vi "LDT1001 Getting Started.vi"(7 "RS485 Addr. (128: RS232)":u32=128 max=128, 9 "Reset / Default (T: Both)":bool=TRUE, 10 "ID Query (T: Check)":bool=TRUE, 11 "Serial Port (Com 1: Default)":u16(ring) items=["Com 1", "Com 2", "Com 3", "Com 4"]) -> (0 "error out":errorcluster, 2 "Instrument Identity":string)   [LabVIEW 2011]
doc: "This VI demonstrates the general use of the instrument VIs. It should operate properly with all series of instruments, namely E2xx, E3xx (new and older revisions), RE3xx and Integra. Since this VI checks for functions supported with every of the instruments, no serious problems should appear.\n\nOnly two instrument dependent errors may appear: 1) if an external circuit is supported but no external sensor is present, 2) if a refrigerator level (i.e. 2) is used, that is not valid for the type of instrument used. For Series Integra automatically the refrigerator level and the pump power level settings are ignored by this Getting started VI.\n\nAll other errors, that may appear, are communication errors.\n\nSo, on any errors, check for proper settings of the communication port, the baudrate and/or the correct RS485 address (or 128 for RS232 communication) first."
panel:
  out "Ramp Programs Message":string="Max. Count of Ramp Programs and Segments is:"
  out "Max. Segment Count":u8
  out "Ramps available":u8
  out "Pump Pressure is (Integra only)":dbl format="%.2f"
  out "External Bath Temperature is:":dbl format="%.2f"
  out "PID Value P/°C":dbl format="%.2f"
  out "PID Value I/s":i32
  out "Upper Temperature":dbl format="%.2f"
  out "Lower Temperature":dbl format="%.2f"
  out "Ext. Circuit Message":string="External Circuit Settings are:"
  out "Error Status Word":string
  out "Software Rev.":string
  out "Hardware Rev.":string
  out "Self-Test":string
  out "Support Message":string="Pump Power / Refrigerator Levels are:"
  in  "Baud Rate (2: 9600 Default)":u16(ring)=2 items=["2400", "4800", "9600", "19200"]
  out "Serial Port":string
  out "PID Value I/s":i32
  out "PID Value P/°C":dbl format="%.2f"
  out "Pump Power Level":u8
  out "Refrigerator Level":u8
  out "Cutoff/°C":dbl format="%.2f"
  out "Bath temperature/°C":dbl format="%.2f"
  out "Setpoint/°C":dbl format="%.2f"
  in  "Setpoint/°C (20.00 °C: Default)":sgl=20.0 min=-35 max=250 step=1 format="%.2f"
  in  "Refrigerator Level (0: Default)":u8 max=3
  in  "Pump Power Level (2: Default)":u8=1 min=1 max=5
  out "Error Message":string="No Error"
  # "Getting Started"
  # "Settings"
  # "Readings"
  # "Communication"
  # "Instrument"
  # "Outlet Temperature Values are:"
  # "Temperature (Primary Circuit Settings) are:"
  # "PID Values External are:"
  # "Check\nDon't Check"
  # "Reset and Default\nDefault only"
  # "PID Values Internal are:"
  # "Instrument"
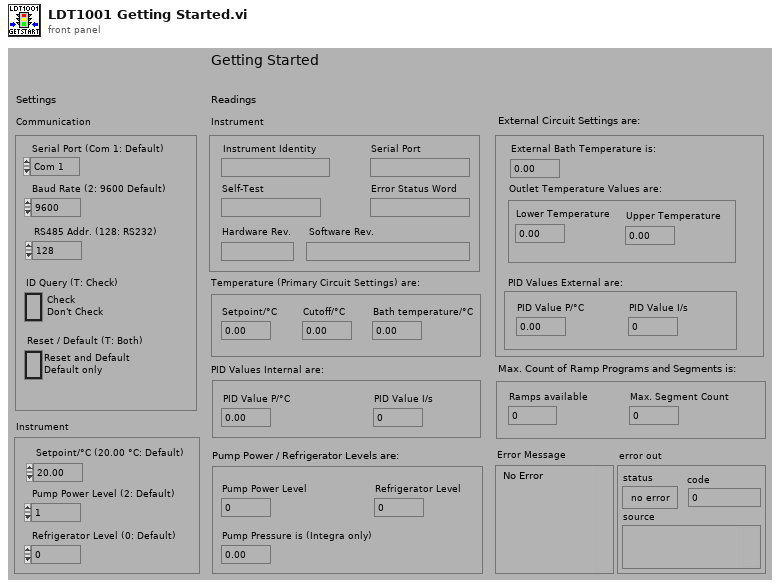
[diagram p1: front panel]
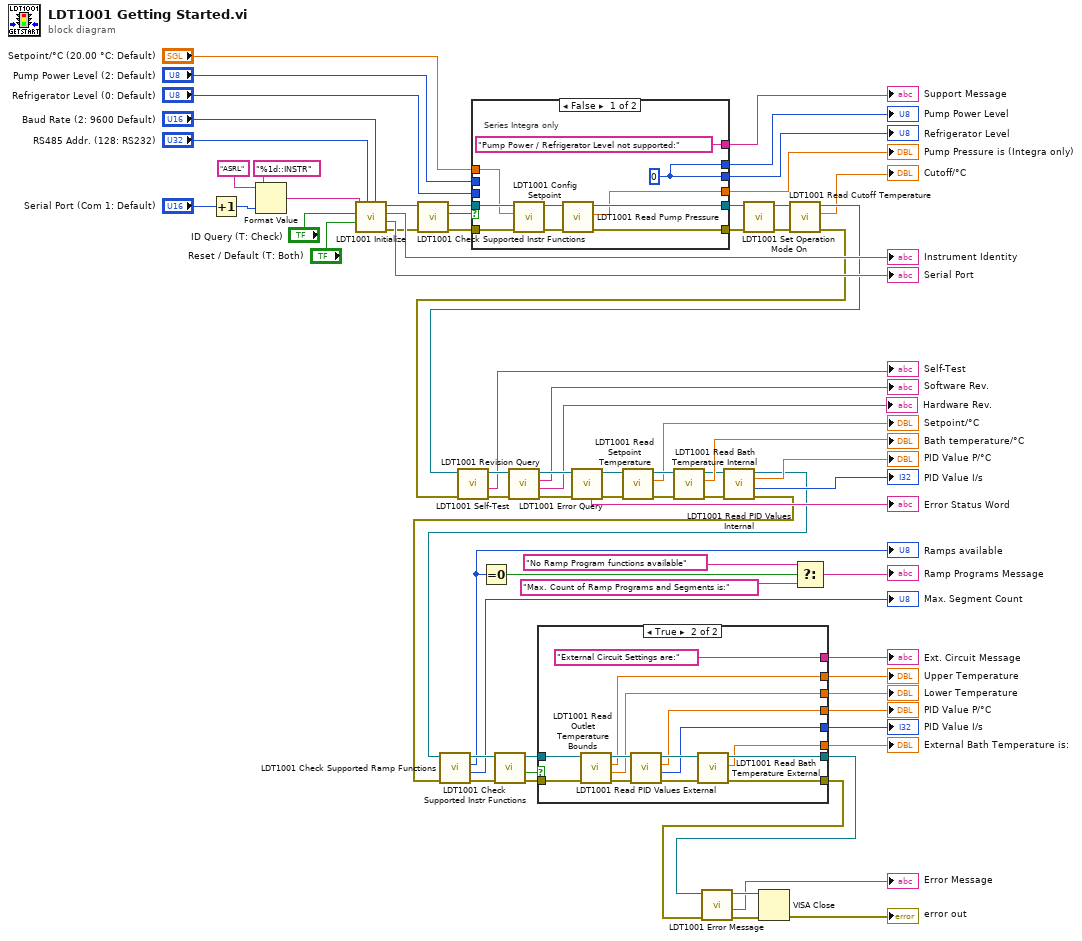
[diagram p0: block diagram]
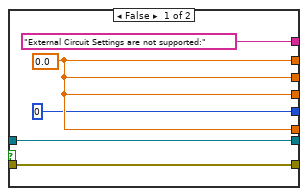
[diagram p2: hidden frame]
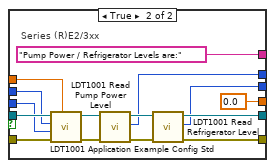
[diagram p3: hidden frame]
diagram:
  n1 = Increment(x="Serial Port (Com 1: Default)") -> (x+1=w53:u16)
  n2 = Format Value(string ("")="ASRL", format string="%1d::INSTR", value (0)=w53) -> (output string=w56:string)
  n3 = call <instrlib>:"LDT1001 Initialize.vi"("Baud Rate (2: 9600 default)"="Baud Rate (2: 9600 Default)", "RS485 Instrument Address (128: RS232 default)"="RS485 Addr. (128: RS232)", "Reset / Default (T: Both)"="Reset / Default (T: Both)", "ID Query (T: Check)"="ID Query (T: Check)", "Instrument Descriptor (ASRL1::INSTR)"=w56) -> ("error out"=w46:errorcluster, "Serial Port"=→"Serial Port":string, "Instrument Identity"=→"Instrument Identity":string, "VISA session"=w47:refnum<visa-resource-name>)  [unwired: 3 in]
  n4 = call <instrlib>:"LDT1001 Check Supported Instr Functions.vi"("error in (no error)"=w46, "VISA session"=w47) -> ("error out"=w49:errorcluster, "Pump/Refrig supported"=w45:bool, "dup VISA session"=w48:refnum<visa-resource-name>)  [unwired: 6 in, 1 out]
  n5 = case shown="False" w45 {
    tunnel: w48 -> [w83 w98]
    tunnel: w49 -> [w82 w97]
    tunnel: [w75 w89] -> w50
    tunnel: [w76 w88] -> w51
    tunnel: "Refrigerator Level (0: Default)" -> [_ w96]
    tunnel: "Pump Power Level (2: Default)" -> [_ w95]
    tunnel: "Setpoint/°C (20.00 °C: Default)" -> [w81 w94]
    tunnel: [w79 w87] -> w41
    tunnel: [w79 w86] -> w65
    tunnel: ["Pump Power / Refrigerator Level not supported:" "Pump Power / Refrigerator Levels are:"] -> w40
    tunnel: [w74 0.0] -> w13
    frame False {
      w79 = u8 0
      # "Series Integra only"
      n6 = call <instrlib>:"LDT1001 Config Setpoint.vi"("error in (no error)"=w82, "Setpoint (20.00 °C: Default)"=w81, "VISA session"=w83) -> ("error out"=w78:errorcluster, "dup VISA session"=w77:refnum<visa-resource-name>)  [unwired: 7 in]
      n7 = call <instrlib>:"LDT1001 Read Pump Pressure.vi"("error in (no error)"=w78, "VISA session"=w77) -> ("error out"=w75:errorcluster, "Pump Pressure"=w74:dbl, "dup VISA session"=w76:refnum<visa-resource-name>)  [unwired: 7 in]
    }
    frame True {
      # "Series (R)E2/3xx"
      n8 = call <instrlib>:"LDT1001 Application Example Config Std.vi"("Setpoint (20.00 °C: Default)"=w94, "error in (no error)"=w97, "Refrigerator Level (0: Default)"=w96, "Pump Power Level (2: Default)"=w95, "VISA session"=w98) -> ("error out"=w90:errorcluster, "dup VISA session"=w92:refnum<visa-resource-name>)  [unwired: 5 in]
      n9 = call <instrlib>:"LDT1001 Read Pump Power Level.vi"("error in (no error)"=w90, "VISA session"=w92) -> ("error out"=w91:errorcluster, "Pump Power Level"=w86:u8, "dup VISA session"=w93:refnum<visa-resource-name>)  [unwired: 7 in]
      n10 = call <instrlib>:"LDT1001 Read Refrigerator Level.vi"("error in (no error)"=w91, "VISA session"=w93) -> ("error out"=w89:errorcluster, "Refrigerator Level"=w87:u8, "dup VISA session"=w88:refnum<visa-resource-name>)  [unwired: 7 in]
    }
  }
  "Pump Power Level" <- w65
  "Refrigerator Level" <- w41
  "Support Message" <- w40
  "Pump Pressure is (Integra only)" <- w13
  n11 = call <instrlib>:"LDT1001 Set Operation Mode On.vi"("error in (no error)"=w50, "VISA session"=w51) -> ("error out"=w25:errorcluster, "dup VISA session"=w24:refnum<visa-resource-name>)  [unwired: 8 in]
  n12 = call <instrlib>:"LDT1001 Read Cutoff Temperature.vi"("error in (no error)"=w25, "VISA session"=w24) -> ("error out"=w26:errorcluster, "Cutoff Temperature"=→"Cutoff/°C":dbl, "dup VISA session"=w27:refnum<visa-resource-name>)  [unwired: 7 in]
  n13 = call <instrlib>:"LDT1001 Self-Test.vi"("error in (no error)"=w26, "VISA session"=w27) -> ("error out"=w36:errorcluster, "Self-Test Response"=→"Self-Test":string, "dup VISA session"=w37:refnum<visa-resource-name>)  [unwired: 6 in, 1 out]
  n14 = call <instrlib>:"LDT1001 Revision Query.vi"("error in (no error)"=w36, "VISA session"=w37) -> ("error out"=w34:errorcluster, "Instr Firmware Revision"=→"Hardware Rev.":string, "Instr Driver Revision"=→"Software Rev.":string, "dup VISA session"=w35:refnum<visa-resource-name>)  [unwired: 6 in]
  n15 = call <instrlib>:"LDT1001 Error Query.vi"("error in (no error)"=w34, "VISA session"=w35) -> ("error out"=w32:errorcluster, "dup VISA session"=w33:refnum<visa-resource-name>, "Error Status Word"=→"Error Status Word":string)  [unwired: 5 in, 2 out]
  n16 = call <instrlib>:"LDT1001 Read Setpoint Temperature.vi"("error in (no error)"=w32, "VISA session"=w33) -> ("error out"=w69:errorcluster, "Setpoint Temperature"=→"Setpoint/°C":dbl, "dup VISA session"=w68:refnum<visa-resource-name>)  [unwired: 7 in]
  n17 = call <instrlib>:"LDT1001 Read Bath Temperature Internal.vi"("error in (no error)"=w69, "VISA session"=w68) -> ("error out"=w38:errorcluster, "Internal Bath Temperature"=→"Bath temperature/°C":dbl, "dup VISA session"=w39:refnum<visa-resource-name>)  [unwired: 7 in]
  n18 = call <instrlib>:"LDT1001 Read PID Values Internal.vi"("error in (no error)"=w38, "VISA session"=w39) -> ("error out"=w10:errorcluster, "Internal PID Value I/s"=→"PID Value I/s":i32, "Internal PID Value P/°C"=→"PID Value P/°C":dbl, "dup VISA session"=w9:refnum<visa-resource-name>)  [unwired: 6 in]
  n19 = call <instrlib>:"LDT1001 Check Supported Ramp Functions.vi"("error in (no error)"=w10, "VISA session"=w9) -> ("error out"=w11:errorcluster, "Max. Segment Count available"=→"Max. Segment Count":u8, "Ramp Programs available"=w7:u8, "dup VISA session"=w12:refnum<visa-resource-name>)  [unwired: 6 in]
  "Ramps available" <- w7
  n20 = Equal To 0?(x=w7) -> (x = 0?=w6:bool)
  n21 = call <instrlib>:"LDT1001 Check Supported Instr Functions.vi"("error in (no error)"=w11, "VISA session"=w12) -> ("error out"=w21:errorcluster, "Ext. Control supported"=w20:bool, "dup VISA session"=w22:refnum<visa-resource-name>)  [unwired: 6 in, 1 out]
  n22 = case shown="True" w20 {
    tunnel: [w99 w117] -> w1
    tunnel: [w100 w116] -> w2
    tunnel: w21 -> [w99 w115]
    tunnel: w22 -> [w100 w112]
    tunnel: ["External Circuit Settings are not supported:" "External Circuit Settings are:"] -> w19
    tunnel: [w102 w108] -> w18
    tunnel: [w102 w107] -> w17
    tunnel: [w102 w106] -> w16
    tunnel: [0 w105] -> w15
    tunnel: [w102 w104] -> w14
    frame False {
      w102 = 0.0
    }
    frame True {
      n23 = call <instrlib>:"LDT1001 Read Outlet Temperature Bounds.vi"("error in (no error)"=w115, "VISA session"=w112) -> ("error out"=w113:errorcluster, "Outlet Lower Temperature"=w107:dbl, "Outlet Upper Temperature"=w108:dbl, "dup VISA session"=w110:refnum<visa-resource-name>)  [unwired: 6 in]
      n24 = call <instrlib>:"LDT1001 Read PID Values External.vi"("error in (no error)"=w113, "VISA session"=w110) -> ("error out"=w114:errorcluster, "External PID Value I/s"=w105:i32, "External PID Value P/°C"=w106:dbl, "dup VISA session"=w111:refnum<visa-resource-name>)  [unwired: 6 in]
      n25 = call <instrlib>:"LDT1001 Read Bath Temperature External.vi"("error in (no error)"=w114, "VISA session"=w111) -> ("error out"=w117:errorcluster, "External Bath Temperature"=w104:dbl, "dup VISA session"=w116:refnum<visa-resource-name>)  [unwired: 6 in, 1 out]
    }
  }
  "Ext. Circuit Message" <- w19
  "Lower Temperature" <- w17
  "Upper Temperature" <- w18
  "PID Value I/s" <- w15
  "PID Value P/°C" <- w16
  "External Bath Temperature is:" <- w14
  n26 = call <instrlib>:"LDT1001 Error Message.vi"("error in (no error)"=w1, "VISA session"=w2) -> ("error out"=w61:errorcluster, "Error Message (empty)"=→"Error Message":string, "dup VISA session"=w62:refnum<visa-resource-name>)  [unwired: 5 in, 2 out]
  n27 = VISA Close(VISA resource name=w62, error in (no error)=w61) -> (error out=→"error out":errorcluster)
  n28 = Select(t="No Ramp Program functions available", s=w6, f="Max. Count of Ramp Programs and Segments is:") -> (s? t:f=→"Ramp Programs Message":string)
